vi "Write Wash Step Indicator.vi"(8 "error in (no error)":errorcluster, 10 "Wash Steps":T1, 11 "Sim Wash Display Console in":refnum<class "Sim Wash Display Console.lvclass">) -> (0 "error out":errorcluster, 3 "Sim Wash Display Console out":refnum<class "Sim Wash Display Console.lvclass">)   [LabVIEW 2019, in "Sim Wash Display Console.lvlib" / "Sim Wash Display Console.lvclass"]
uses:
  Sim Wash Display Console.lvclass
  Car Wash Controller/Car Wash Controller/Wash Steps.ctl
  Car Wash Controller/Car Wash Controller/Car Wash Controller.lvclass
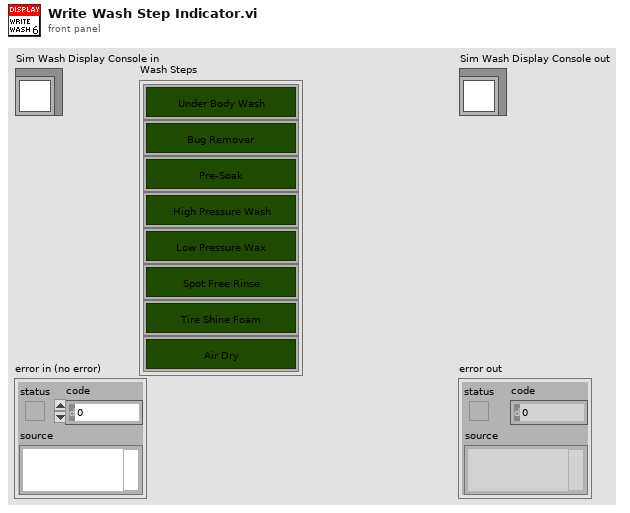
[diagram p1: front panel]
types:
  T1 = typedef "Car Wash Controller.lvlib/Car Wash Controller.lvclass/Wash Steps.ctl" = cluster{"Under Body Wash":bool, "Bug Remover":bool, "Pre-Soak":bool, "High Pressure Wash (Default)":bool, "Low Pressure Wax":bool, "Spot Free Rinse":bool, "Tire Shine Foam":bool, "Air Dry":bool}
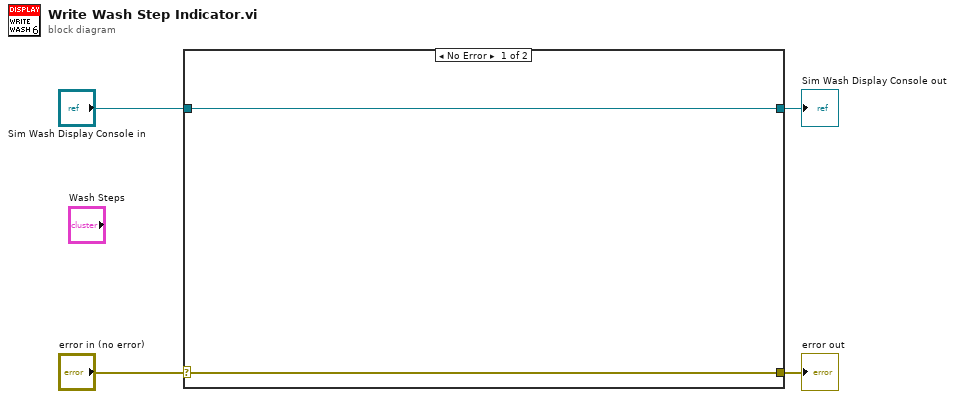
[diagram p0: block diagram]
diagram:
  n1 = case shown="No Error" "error in (no error)" {
    selector: "error in (no error)" -> [w6 w8]
    tunnel: [w6 w8] -> w3
    tunnel: [w5 w7] -> w1
    tunnel: "Sim Wash Display Console in" -> [w5 w7]
    frame No Error {
    }
    frame Error {
    }
  }
  "error out" <- w3
  "Sim Wash Display Console out" <- w1
